vi "Status.TEST - Simple LED Status Indicator.vi"() -> ()   [LabVIEW 2024, in "EQMF.lvlib" / "Status Utils.lvlib"]
uses:
  Status Utils.lvlib
panel:
  in  "Show OK":bool
  in  "Blink":bool
  in  "stop":bool
  in  "error in (no error)":errorcluster
  out "Boolean 2":bool
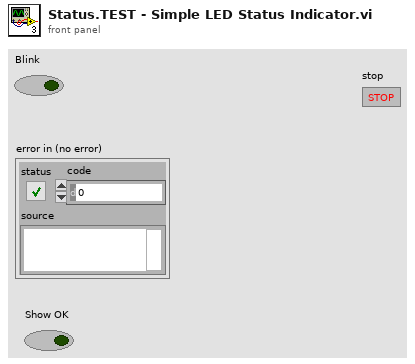
[diagram p1: front panel]
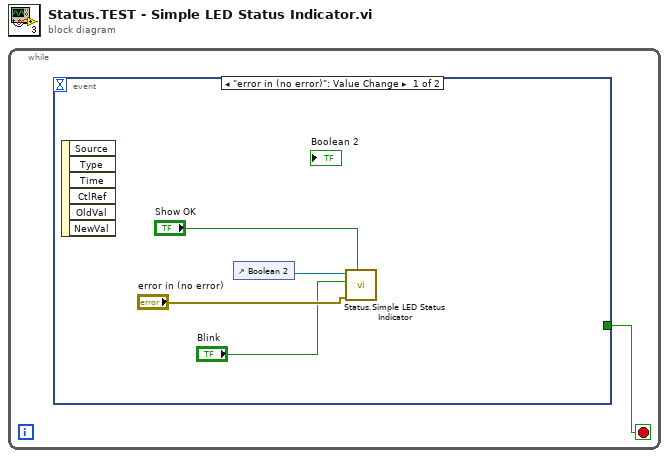
[diagram p0: block diagram]
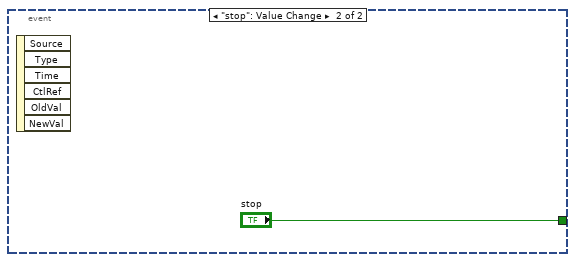
[diagram p2: hidden frame]
diagram:
  n1 = while {
    stop <- w1 stop-if-true
    n2 = event shown="[0] \"error in (no error)\": Value Change" {
      selector: _ -> [_ _]
      dyn-events: _ -> [_ _]
      timeout: _ -> [_ _]
      tunnel: [_ "stop"] -> w1
      event "error in (no error)": Value Change {
        n3 = event-data() -> ()  [unwired: 1 in, 6 out]
        n4 = control-ref of="Boolean 2"() -> (w5:refnum<vi>)
        n5 = call "Status.Simple LED Status Indicator.vi"("Show OK Indication"="Show OK", "error in"="error in (no error)", "Blink on Error"="Blink", "LED Status"=w5) -> ()  [unwired: 7 in, 1 out]
      }
      event "stop": Value Change {
        n6 = event-data() -> ()  [unwired: 1 in, 6 out]
      }
    }
  }
